vi "obtain GFG_core VI Ref.vi"(11 "file path (use dialog)":path) -> (3 "GFG_core VI ref out":refnum<vi>)   [LabVIEW 2012, in "GFG library.lvlib"]
uses:
  GFG library.lvlib
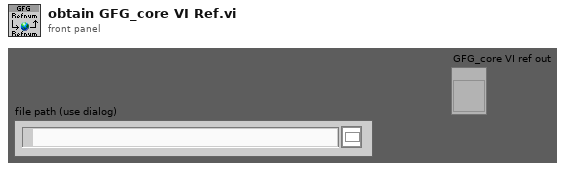
[diagram p1: front panel]
types:
  T1 = enum16{"open", "replace", "create", "open or create", "replace or create", "replace or create with confirmation"}
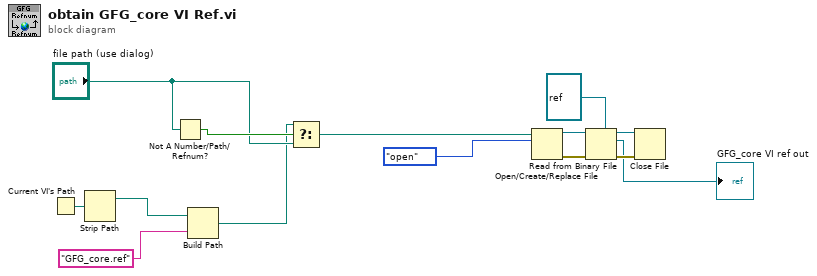
[diagram p0: block diagram]
diagram:
  n1 = Current VI's Path() -> (path=w7:path)
  n2 = Strip Path(path=w7) -> (stripped path=w6:path)  [unwired: 1 out]
  n3 = Not A Number/Path/Refnum?(number/path/refnum="file path (use dialog)") -> (NaN/Path/Refnum?=w4:bool)
  n4 = Build Path(base path=w6, name or relative path="GFG_core.ref" ("replace string (\"\")")) -> (appended path=w2:path)
  n5 = Select(t=w2, s=w4, f="file path (use dialog)") -> (s? t:f=w1:path)
  n6 = Open/Create/Replace File(file path (use dialog)=w1, operation (0:open)=T1."open") -> (refnum out=w12:refnum<file>, error out=w13:errorcluster)  [unwired: 4 in, 1 out]
  n7 = Read from Binary File(5:refnum<vi> refnum ("type specifier VI Refnum (for type only)"), 8:w13, 11:w12) -> (0:w10:errorcluster, 2:→"GFG_core VI ref out":refnum<vi>, 3:w11:refnum<file>)  [unwired: 3 in, 1 out]
  n8 = Close File(refnum=w11, error in=w10) -> ()  [unwired: 2 out]
